vi "Start Test.vi"(8 "error in (no error)":errorcluster, 11 "Start Test":bool) -> (0 "error out":errorcluster, 3 "Connection Established?":bool)   [LabVIEW 2019]
doc: "Establishes connection between client and server"
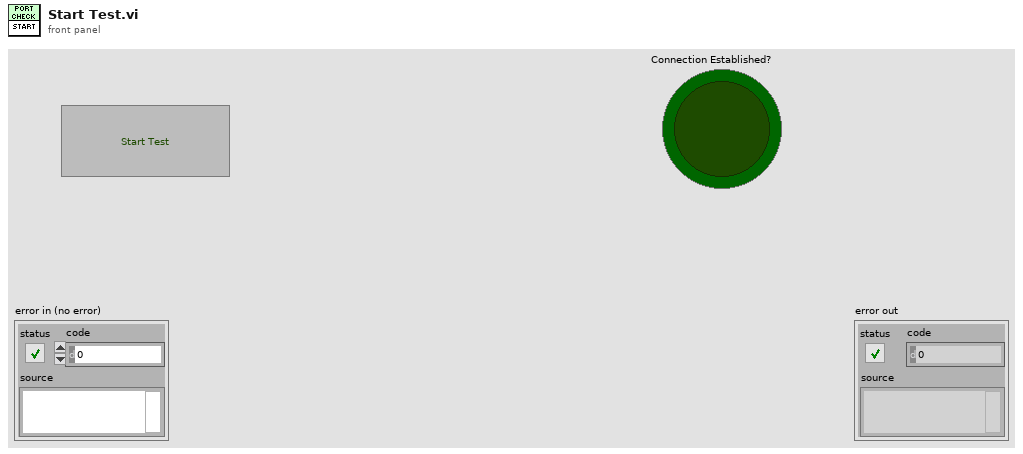
[diagram p1: front panel]
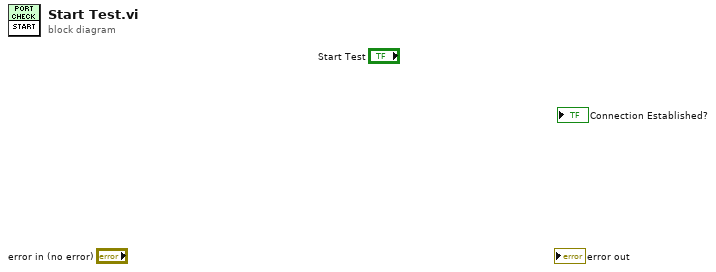
[diagram p0: block diagram]
diagram:
